vi "PhysiologyExperiment.vi"() -> ()   [LabVIEW 2017]
doc: "I. Description:\nThis example demonstrates how to continuously acquire and generate data at the same time, synchronized with one another.\n\nII. Instructions for Running:\n1. Select the physical channel to correspond to where your signal is input on the DAQ device. Also, select the corresponding channel for where your signal is being generated.\n2. Enter the minimum and maximum voltage ranges.\nNote: For better accuracy try to match the input range to the expected voltage level of the measured signal.\n3. Set the sample rate of the acquisition.\nNote: The rate should be at least twice as fast as the maximum frequency component of the signal being acquired. \n4. Select the Rate for the generation\n5. Select what type of signal to generate and the amplitude.\nNote: This example requires two DMA channels to run. If your hardware does not support two DMA channels, you need to set the Data Transfer Mechanism property for the Analog Output Task to use \"Interrupts\". The Data Transfer Mechanism property is located in the DAQmx Channel Property hierarchy at: DAQmx Channel Property Node>>Analog Output>>General Properties>>Advanced>>Data Transfer and Memory>>Data Transfer Mechanism\n\nRefer to your device documentation to determine how many DMA channels are supported for your hardware.\n\nIII. Block Diagram Steps:\n1. Create an analog input voltage channel. Also, create an analog output voltage channel.\n2. Set the rate for the sample clock. Additionally, define the sample mode to be continuous. Also, set the sample clock rate for the signal generation.\n2a. Call the Get Terminal Name with Device Prefix VI. This will take a Task and a terminal and create a properly formatted device + terminal name to use as the source of the Trigger.\n3. Define the parameters for a Digital Edge Start Trigger. Set the Analog output to trigger off the AI Start Trigger. This is an internal trigger signal.\n4. Use the Basic Function Generator VI to create the signal to be generated.\n5. Call the Start VI to arm the two functions. Make sure the analog output is armed before the analog input. This will ensure both will start at the same time.\n6. Read the waveform data in a loop until the user hits the stop button or an error occurs. The Is Task Done? VI is used to check for errors in the Analog Output Task.\n7. Call the Clear VI to Clear the Task\n8. Use the popup dialog box to display an error if any.\n\nIV. I/O Connections Overview:\nMake sure your signal input/output terminals match the Physical Channel I/O controls."
uses:
  <vilib>/Utility/error.llb/DialogType.ctl
panel:
  in  "External trigger (PFI0) (if true, minimum stim interval is ignored)":bool
  in  "Minimum Stim Interval (s)":dbl=2.0
  in  "Filter type":u16(ring) items=["no filter", "4k high-pass filter", "4k-20k band-pass", "4k-50k band-pass"]
  out "Stimulus time remaining (min)":dbl
  in  "Stimulus multipliers (comma sep.)":string="0.1, 1, 10"
  out "Current multiplier":dbl
  in  "Stimulus folder":path=path "C:/data/Auditory/gen5/fullfield"
  out "Number of files Remaining":dbl
  out "Current stimulus file":string
  out "Number of stim files":dbl
  out "Number of multipliers":dbl
  out "Current stimulus overview":waveform(dbl)[](graph)
  out "Digital Waveform Graph":digitalwaveform(graph) caption="TTL pulses"
  # "Overview: This VI Generates Synchronized 2ch auditory stimulation and synchronization pulses\nRequirements: \nSoftware: LabVIEW 2012 (or compatible). The digital port need to support buffered operations (port 0 on PCIe-6341)\nInstructions: \n1. Choose the stimulus folder that contains multiple .wav files )\n2.\tSet mulitpliers in by comma separated numbers\n3. Start stimuli\nNotes:\nEach .wav should be ~1 min or less at 500 kHz, and should be 16-bit integer format with 3 channels (3rd channel contains TTL pulses).\nRemaining time is valid only if stim files have the same durations."
  # "Stimulus control"
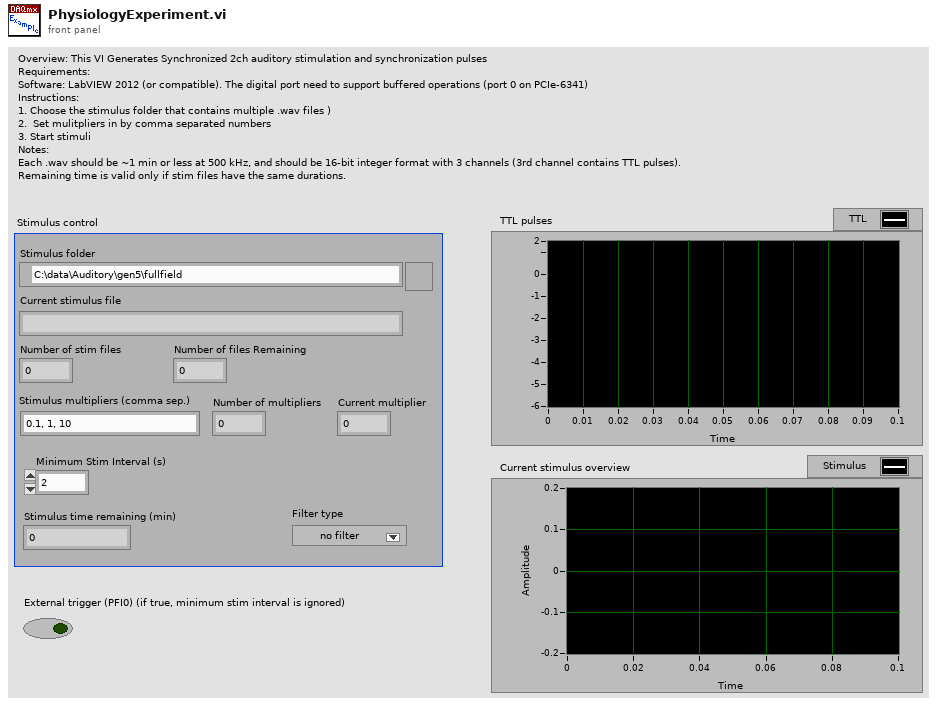
[diagram p1: front panel]
types:
  T1 = enum16{"open", "replace", "create", "open or create", "replace or create", "replace or create with confirmation"}
  T2 = typedef "DialogType.ctl" = u16
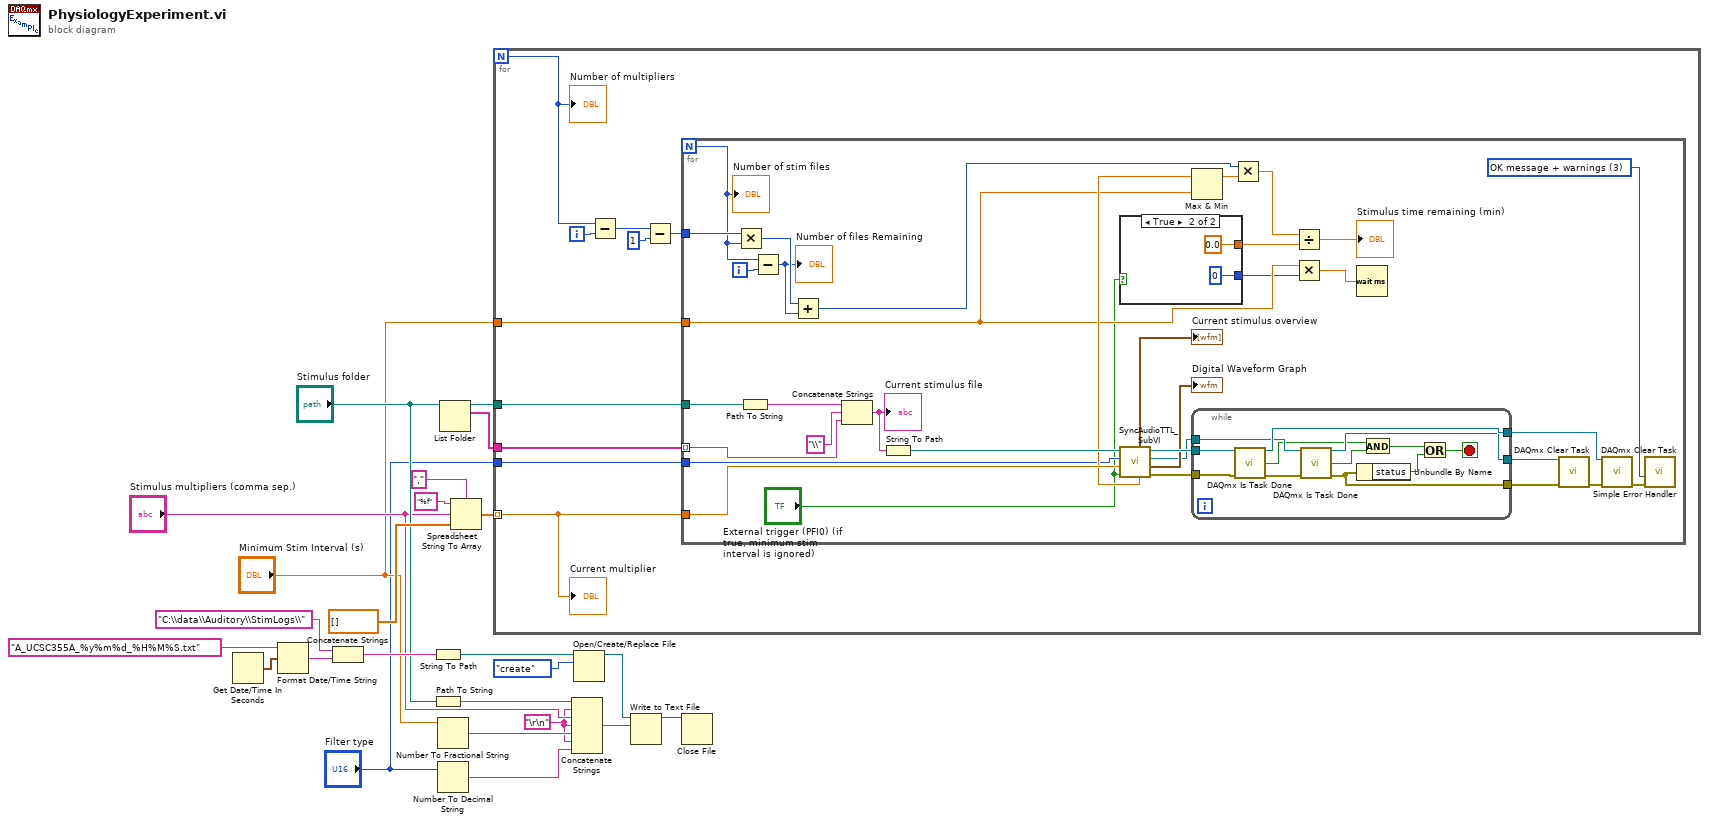
[diagram p0: block diagram]
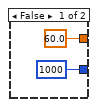
[diagram p2: hidden frame]
diagram:
  w5 = "\r\n"
  n1 = Get Date/Time In Seconds() -> (seconds since 1Jan1904=w18:timestamp)
  n2 = Format Date/Time String(time format string (%c)="A_UCSC355A_%y%m%d_%H%M%S.txt", seconds (now)=w18) -> (date/time string=w17:string)  [unwired: 1 in]
  n3 = Concatenate Strings("C:\\data\\Auditory\\StimLogs\\", w17) -> (w15:string)
  n4 = String To Path(string=w15) -> (path=w14:path)
  n5 = Path To String(path="Stimulus folder") -> (string=w8:string)
  n6 = Number To Fractional String(number="Minimum Stim Interval (s)") -> (F-format string=w6:string)  [unwired: 3 in]
  n7 = Number To Decimal String(number="Filter type") -> (decimal integer string=w3:string)  [unwired: 1 in]
  n8 = List Folder(path="Stimulus folder") -> (path out=w10:path, filenames=w11:string[])  [unwired: 3 in, 2 out]
  n9 = Spreadsheet String To Array(delimiter (Tab)=",", format string="%f", spreadsheet string="Stimulus multipliers (comma sep.)", array type (2D Dbl)=dbl[] []) -> (array=w21:dbl[])
  n10 = for {
    N -> [w32]
    tunnel: w21 -> [w34] mode=indexing
    tunnel: w11 -> [w28]
    tunnel: w10 -> [w27]
    tunnel: "Minimum Stim Interval (s)" -> [w26]
    tunnel: "Filter type" -> [w25]
    i -> [w33]
    n11 = Subtract(x=w32, y=w33) -> (x-y=w30:i32)
    n12 = Subtract(x=w30, y=1) -> (x-y=w29:i32)
    n13 = for {
      N -> [w50]
      tunnel: w34 -> [w54]
      tunnel: w29 -> [w51]
      tunnel: w28 -> [w41] mode=indexing
      tunnel: w27 -> [w40]
      tunnel: w26 -> [w39]
      tunnel: w25 -> [w38]
      i -> [w66]
      w55 = T2 3 items=["no dialog", "OK message", "continue or stop message", "OK message + warnings", "continue/stop + warnings"] ("type of dialog (OK msg:1)")
      n14 = Multiply(x=w51, y=w50) -> (x*y=w49:i32)
      n15 = Path To String(path=w40) -> (string=w68:string)
      n16 = Subtract(x=w50, y=w66) -> (x-y=w48:i32)
      "Number of files Remaining" <- w48
      n17 = Add(x=w49, y=w48) -> (x+y=w42:i32)
      n18 = Concatenate Strings(w68, "\\", w41) -> (w53:string)
      "Current stimulus file" <- w53
      n19 = String To Path(string=w53) -> (path=w52:path)
      n20 = case shown="True" "External trigger (PFI0) (if true, minimum stim interval is ignored)" {
        tunnel: [1000 0] -> w36
        tunnel: [60.0 0.0] -> w35
        frame False {
        }
        frame True {
        }
      }
      n21 = call "SyncAudioTTL_SubVI.vi"("External Trigger"="External trigger (PFI0) (if true, minimum stim interval is ignored)", "Multiplier"=w54, "Filter Type"=w38, "Stimulus File"=w52) -> ("error out"=w65:errorcluster, "digital waveform"=→"Digital Waveform Graph":digitalwaveform, "task out 2"=w57:refnum<k21>, "Refnum out"=w64:refnum<k21>, "Stim File Length (s)"=w44:dbl, "Array"=→"Current stimulus overview":waveform(dbl)[])  [unwired: 2 in]
      n22 = Max & Min(x=w44, y=w39) -> (max(x,y)=w43:dbl)  [unwired: 1 out]
      n23 = while {
        tunnel: [w84] -> w56
        tunnel: w57 -> [w82]
        tunnel: [w81] -> w58
        tunnel: [w80] -> w59
        tunnel: w64 -> [w75]
        tunnel: w65 -> [w74]
        stop <- w76 stop-if-true
        n24 = call <vilib>:"DAQmx Is Task Done.vi"("task/channels in"=w75, "error in"=w74) -> ("task out"=w84:refnum<k21>, "task done?"=w79:bool, "error out"=w83:errorcluster)  [unwired: 2 in, 9 out]
        n25 = call <vilib>:"DAQmx Is Task Done.vi"("task/channels in"=w82, "error in"=w83) -> ("task out"=w81:refnum<k21>, "task done?"=w78:bool, "error out"=w80:errorcluster)  [unwired: 11 out]
        n26 = Unbundle By Name(w80) -> ("status"=w73:bool)
        n27 = And(x=w79, y=w78) -> (x .and. y?=w77:bool)
        n28 = Or(x=w77, y=w73) -> (x .or. y?=w76:bool)
      }
      n29 = Multiply(x=w42, y=w43) -> (x*y=w47:dbl)
      n30 = Divide(x=w47, y=w35) -> (x/y=→"Stimulus time remaining (min)":dbl)
      n31 = Multiply(x=w39, y=w36) -> (x*y=w45:dbl)
      n32 = Wait (ms)(milliseconds to wait=w45) -> ()  [unwired: 1 out]
      n33 = call <vilib>:"DAQmx Clear Task.vi"("task in"=w58, "error in"=w59) -> ("error out"=w60:errorcluster)  [unwired: 13 out]
      n34 = call <vilib>:"DAQmx Clear Task.vi"("task in"=w56, "error in"=w60) -> ("error out"=w63:errorcluster)  [unwired: 13 out]
      n35 = call <vilib>:"Simple Error Handler.vi"("type of dialog (OK msg:1)"=w55, "error in (no error)"=w63) -> ()  [unwired: 3 in, 5 out]
      "Number of stim files" <- w50
    }
    "Current multiplier" <- w34
    "Number of multipliers" <- w32
  }
  n36 = Concatenate Strings(w8, w5, "Stimulus multipliers (comma sep.)", w5, w6, w5, w3) -> (w4:string)
  n37 = Open/Create/Replace File(file path (use dialog)=w14, operation (0:open)=T1."create") -> (refnum out=w13:refnum<file>)  [unwired: 4 in, 2 out]
  n38 = Write to Text File(file (use dialog)=w13, text=w4) -> (refnum out=w12:refnum<file>)  [unwired: 2 in, 2 out]
  n39 = Close File(refnum=w12) -> ()  [unwired: 1 in, 2 out]
